vi "User@TextRingValue__Parameter.vi"(1 "ParamterIn":string) -> (0 "ParamterOut":string)   [LabVIEW 2019]
panel:
  in  "Parameters":string(combo)
  in  "UserPanelControl":string(combo)
  in  "Confirm":bool
  # "User@TextRingValue $UserPanelControlName,$String2Show"
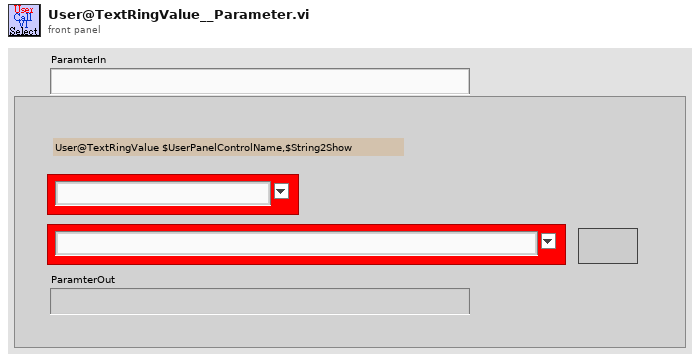
[diagram p1: front panel]
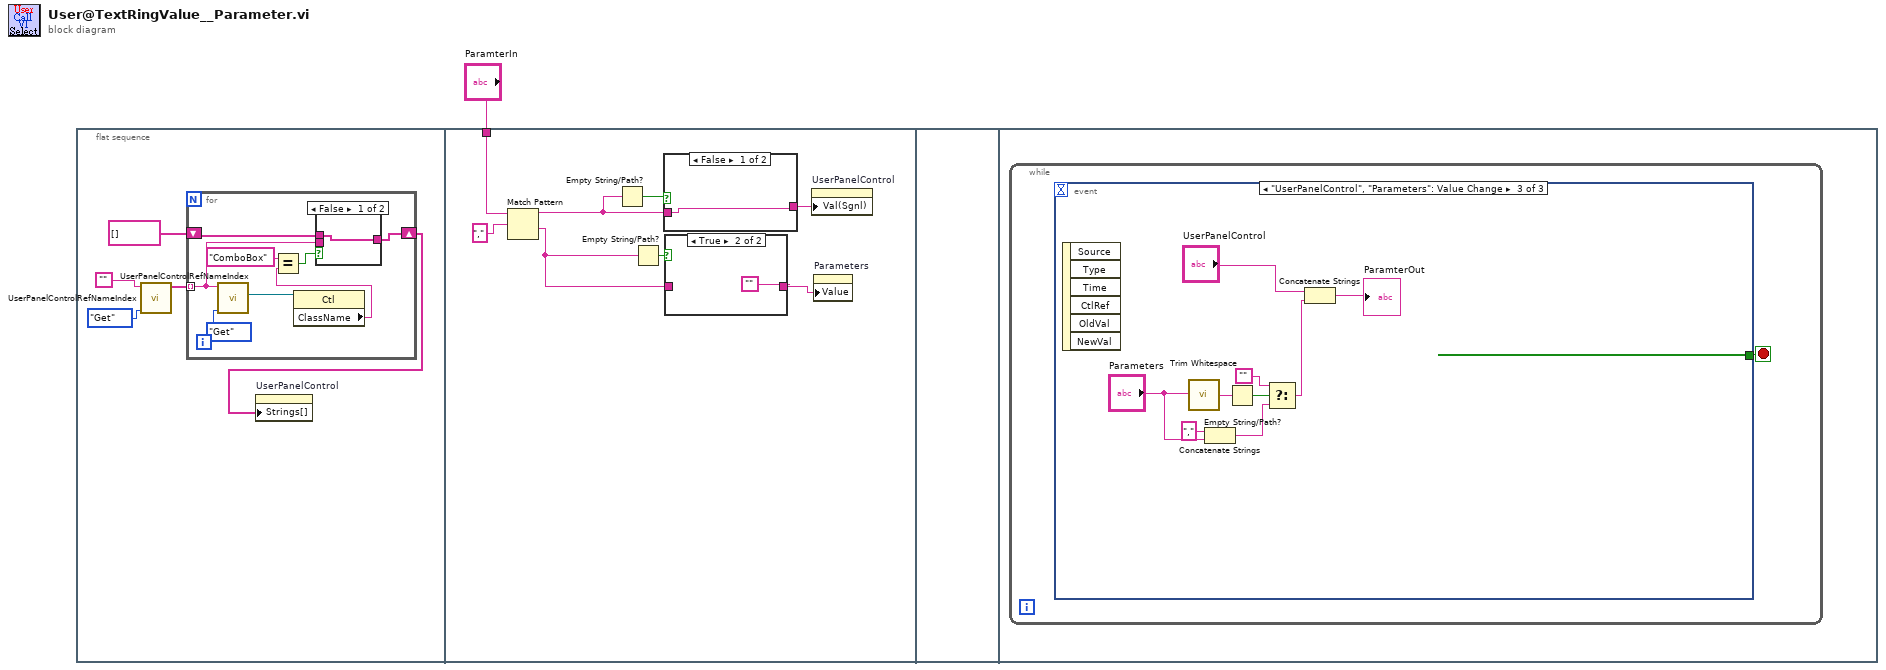
[diagram p0: block diagram]
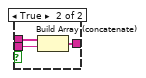
[diagram p2: hidden frame]
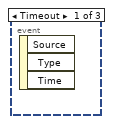
[diagram p5: hidden frame]
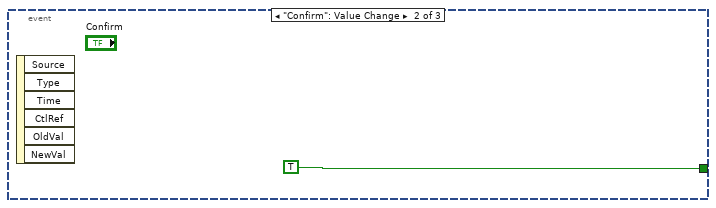
[diagram p6: hidden frame]
diagram:
  n1 = flat-sequence {
    tunnel: "ParamterIn" -> [w24]
    frame #0 {
      n2 = call "UserPanelControlRefNameIndex.vi"("OP"=enum16{"Get", "Update", "Init"}."Get", "ControlName"="") -> ("ControlNameS"=w4:string[])  [unwired: 6 in, 3 out]
      n3 = for {
        tunnel: w4 -> [w9] mode=indexing
        shift-right: [w8] -> w2
        shift-left: string[] [] ("Strings []") -> [w10]
        n4 = call "UserPanelControlRefNameIndex.vi"("OP"=enum16{"Get", "Update", "Init"}."Get", "ControlName"=w9) -> ("ControlRefOut"=w13:refnum<vi>)  [unwired: 6 in, 3 out]
        n5 = property class="Ctl"(reference=w13) -> ("ClassName"=w12:string)  [unwired: 1 in, 2 out]
        n6 = Equal?(x="ComboBox" ("Class Name"), y=w12) -> (x = y?=w11:bool)
        n7 = case shown="False" w11 {
          tunnel: w10 -> [w15 w18]
          tunnel: w9 -> [_ w17]
          tunnel: [w15 w16] -> w8
          frame False {
          }
          frame True {
            n8 = Build Array (concatenate)(w18, w17) -> (w16:string[])
          }
        }
      }
      n9 = property on="UserPanelControl" class="CmbBox"("Strings[]"=w2) -> ()  [unwired: 2 in, 2 out]
    }
    frame #1 {
      n10 = Match Pattern(string=w24, regular expression=",") -> (before substring=w22:string, after substring=w21:string)  [unwired: 1 in, 2 out]
      n11 = Empty String/Path?(string/path=w22) -> (empty?=w26:bool)
      n12 = Empty String/Path?(string/path=w21) -> (empty?=w25:bool)
      n13 = case shown="False" w26 {
        tunnel: w22 -> [w29 w30]
        tunnel: [w29 w30] -> w19
        frame False {
        }
        frame True {
        }
      }
      n14 = case shown="True" w25 {
        tunnel: [w27 ""] -> w20
        tunnel: w21 -> [w27 _]
        frame False {
        }
        frame True {
        }
      }
      n15 = property on="UserPanelControl" class="CmbBox"("Val(Sgnl)"=w19) -> ()  [unwired: 2 in, 2 out]
      n16 = property on="Parameters" class="CmbBox"("Value"=w20) -> ()  [unwired: 2 in, 2 out]
    }
    frame #2 {
    }
    frame #3 {
      n17 = while {
        stop <- w31 stop-if-true
        n18 = event shown="[2] \"UserPanelControl\", \"Parameters\": Value Change" {
          selector: _ -> [_ _ _]
          dyn-events: _ -> [_ _ _]
          timeout: _ -> [_ _ _]
          tunnel: [_ TRUE _] -> w31
          event Timeout {
            n19 = event-data() -> ()  [unwired: 1 in, 3 out]
          }
          event "Confirm": Value Change {
            n20 = event-data() -> ()  [unwired: 1 in, 6 out]
          }
          event "UserPanelControl", "Parameters": Value Change {
            n21 = event-data() -> ()  [unwired: 1 in, 6 out]
            n22 = call <vilib>:"Trim Whitespace.vi"("string"="Parameters") -> ("trimmed string"=w37:string)  [unwired: 1 in]
            n23 = Concatenate Strings("," ("string"), "Parameters") -> (w36:string)
            n24 = Empty String/Path?(string/path=w37) -> (empty?=w38:bool)
            n25 = Select(t="", s=w38, f=w36) -> (s? t:f=w33:string)
            n26 = Concatenate Strings("UserPanelControl", w33) -> (→"ParamterOut":string)
          }
        }
      }
    }
  }
